vi "Actor Core.vi"(8 "error in":errorcluster, 11 "XboxController-V in":refnum<class "XboxController-V.lvclass">) -> (0 "error out":errorcluster, 3 "Actor out":refnum<class "Actor.lvclass">)   [LabVIEW 2013, in "XboxController-V.lvclass"]
doc: "(<B>Filename</B>: Actor Framework.lvlib:Actor.lvclass:Actor Core.vi)\n\nReceives messages to the actor, reacts to them, and initiates any error handling that may shut the actor down.\n\nDescendant classes may override this VI to append parallel tasks for the actor to complete while it handles messages. Overrides use the Call Parent Method node."
uses:
  XboxController-V.lvclass
  <vilib>/ActorFramework/Actor/Actor.lvclass
  XboxController-V.lvclass/XboxController-V.ctl
  Logical Systems/XBoxController/XBoxController.lvclass
panel:
  out "XBox Controller Layout":T1 {"Right Joystick Right" scale=-1.0..1.0; "Left Joystick Right" scale=-1.0..1.0; "Right Joystick Forward" scale=-1.0..1.0; "Left Joystick Forward" scale=-1.0..1.0}
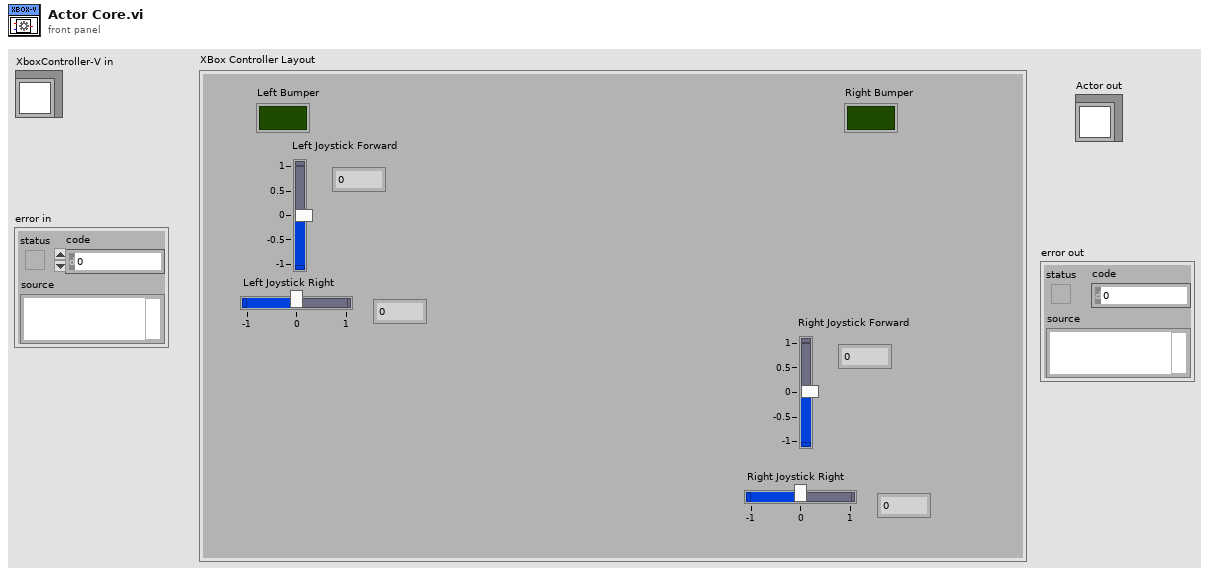
[diagram p1: front panel]
types:
  T1 = cluster{"Left Bumper":bool, "Right Bumper":bool, "Left Joystick Forward":dbl, "Left Joystick Right":dbl, "Right Joystick Forward":dbl, "Right Joystick Right":dbl}
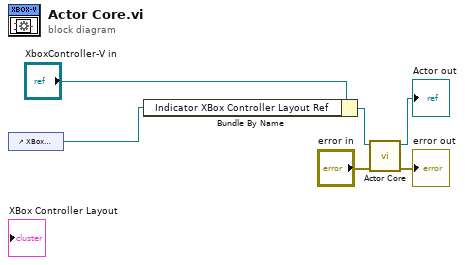
[diagram p0: block diagram]
diagram:
  n1 = control-ref of="XBox Controller Layout"() -> (w1:refnum<vi>)
  n2 = Bundle By Name(cluster="XboxController-V in", "Indicator XBox Controller Layout Ref"=w1) -> (w2:refnum<class "XboxController-V.lvclass">)
  n3 = call-parent "Actor Core.vi"("error in"="error in", "XBoxController in"=w2) -> ("error out"=→"error out":errorcluster, "Actor out"=→"Actor out":refnum<class "Actor.lvclass">)  [unwired: 8 in]
